vi "Auto Fit Width By Col Header.vi"(8 "error in (no error)":errorcluster caption="错误输入（无错误）", 11 "Table Ref In":refnum<vi>) -> (0 "error out":errorcluster caption="错误输出", 3 "Table Ref Out":refnum<vi>)   [LabVIEW 2013, in "Table Tool.lvlib"]
uses:
  Table Tool.lvlib
  Custum Type/Selet Row or Col.ctl
  <vilib>/Utility/miscctls.llb/LVRowAndColumnTypeDef.ctl
  Property/Set Or get Row Head and Column Head Strings.vi
panel:
  in  "Space":i16=20
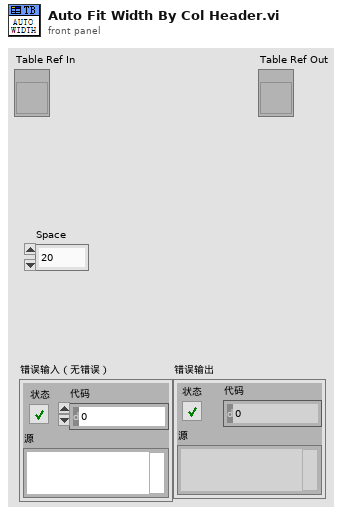
[diagram p1: front panel]
types:
  T1 = typedef "LVRowAndColumnTypeDef.ctl" = cluster{"Row":i32, "Column":i32}
  T2 = typedef "Table Tool.lvlib/Selet Row or Col.ctl" = enum16{"Col", "Row"}
  T3 = cluster{"left":i16, "top":i16, "right":i16, "bottom":i16}
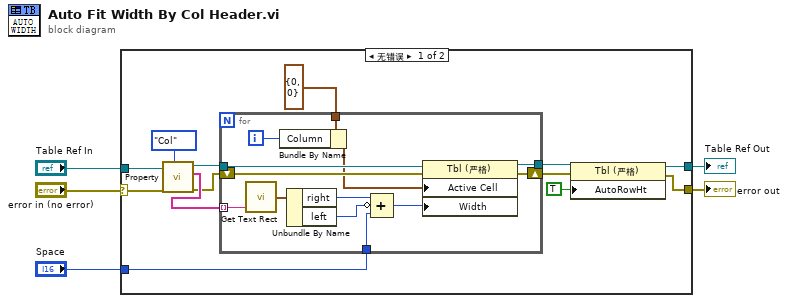
[diagram p0: block diagram]
diagram:
  n1 = case shown="无错误" "error in (no error)" {
    selector: "error in (no error)" -> [w16 w33]
    tunnel: "Table Ref In" -> [w17 w32]
    tunnel: [w8 w32] -> w3
    tunnel: [w7 w33] -> w2
    tunnel: "Space" -> [w14 _]
    frame No Error {
      n2 = call-poly "Property.vi"("Row or Col Option"=Selet_Row_or_Col."Col", "error in (no error)"=w16, "Table Ref In"=w17) -> ("error out"=w12:errorcluster, "Headers[] Out"=w15:string[], "Table Ref Out"=w13:refnum<vi>)  [unwired: 6 in]
      n3 = for {
        tunnel: w15 -> [w31] mode=indexing
        tunnel: w14 -> [w27]
        tunnel: w13 -> [w24]
        shift-right: [w25] -> w10
        shift-left: w12 -> [w26]
        tunnel: [w23] -> w11
        tunnel: T1 {"Row"=0, "Column"=0} ("Active Cell:Active Cell") -> [w21]
        i -> [w20]
        n4 = call <vilib>:"Get Text Rect.vi"("text"=w31) -> ("rect"=w30:T3)  [unwired: 8 in]
        n5 = Bundle By Name(cluster=w21, "Column"=w20) -> (w19:T1)
        n6 = Unbundle By Name(w30) -> ("right"=w29:i16, "left"=w28:i16)
        n7 = Compound Arithmetic op=ADD(w29, invert w28, w27) -> (w22:i16)
        n8 = property class="Tbl (严格)"(reference=w24, error in=w26, "Active Cell"=w19, "Width"=w22) -> (reference out=w23:refnum<vi>, error out=w25:errorcluster)
      }
      n9 = property class="Tbl (严格)"(reference=w11, error in=w10, "AutoRowHt"=TRUE ("自动调整行高")) -> (reference out=w8:refnum<vi>, error out=w7:errorcluster)
    }
    frame Error {
    }
  }
  "Table Ref Out" <- w3
  "error out" <- w2
